vi "solar_qtimer Create.vi"(8 "error in (no error)":errorcluster, 9 "Create if not found? (T)":bool=TRUE, 11 "Interface":string) -> (0 "error out":errorcluster, 3 "QTimer Refnum":T1)   [LabVIEW 2018]
doc: "This creates a QTimer interface that controls all QTimers within a SOLAR application."
uses:
  solar_qtimer_ctl Refnum.ctl
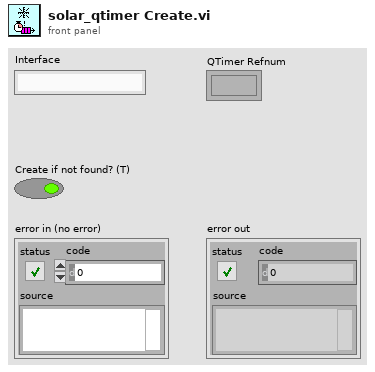
[diagram p1: front panel]
types:
  T1 = typedef "solar_qtimer_ctl Refnum.ctl" = refnum<k1>
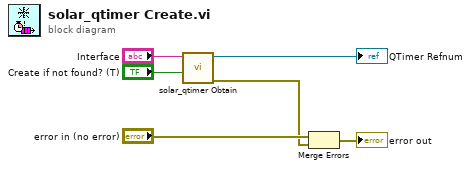
[diagram p0: block diagram]
diagram:
  n1 = call "solar_qtimer Obtain.vi"("Create if not found? (T)"="Create if not found? (T)", "Interface"="Interface") -> ("error out"=w1:errorcluster, "QTimer Refnum"=→"QTimer Refnum":T1)  [unwired: 8 in]
  n2 = Merge Errors("error in (no error)", w1) -> (→"error out":errorcluster)
